vi "M2因子计算.vi"(8 "method":T1 items=["Least Square", "Least Absolute Residual", "Bisquare"], 9 "位置":dbl[](array[numeric]), 10 "光斑半径":dbl[](array[numeric]), 11 "激光波长":dbl) -> (0 "瑞利长度":dbl, 1 "束腰直径":dbl, 2 "束腰位置Z0":dbl, 3 "M2因子":dbl, 4 "光束发散角":dbl)   [LabVIEW 2015]
uses:
  <vilib>/Analysis/6fits.llb/Curve Fitting Criteria.ctl
  <vilib>/Analysis/NI_AALPro.lvlib
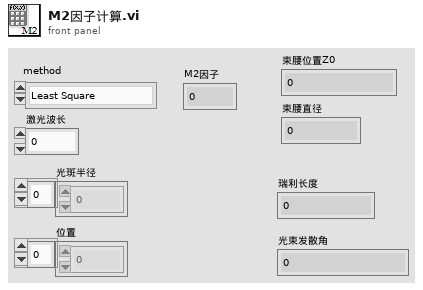
[diagram p1: front panel]
types:
  T1 = typedef "NI_AALPro.lvlib/Curve Fitting Criteria.ctl" = u16
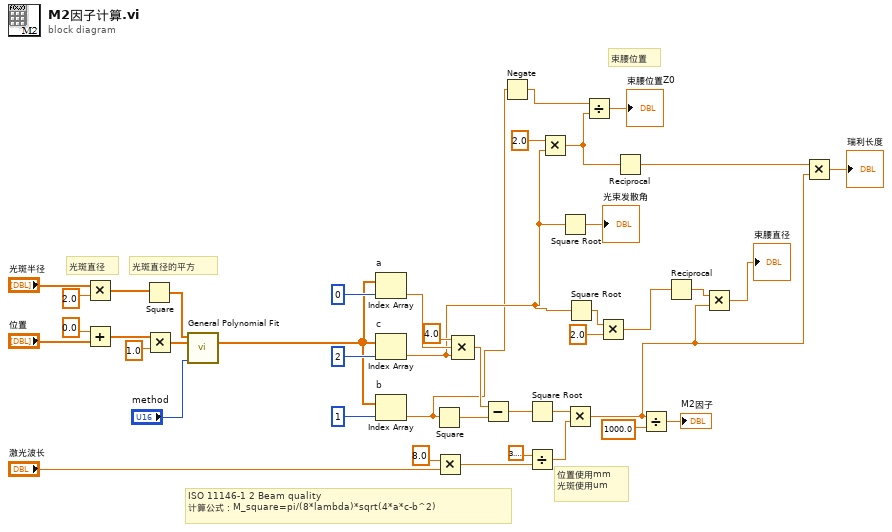
[diagram p0: block diagram]
diagram:
  # "束腰位置"
  # "位置使用mm\n光斑使用um"
  # "ISO 11146-1 2 Beam quality\n计算公式：M_square=pi/(8*lambda)*sqrt(4*a*c-b^2)"
  # "光斑直径的平方"
  # "光斑直径"
  n1 = Multiply(x="光斑半径", y=2.0) -> (x*y=w38:dbl[])
  n2 = Add(x=0.0, y="位置") -> (x+y=w41:dbl[])
  n3 = Square(x=w38) -> (x^2=w37:dbl[])
  n4 = Multiply(x=w41, y=1.0 ("x")) -> (x*y=w36:dbl[])
  n5 = call <vilib>:"General Polynomial Fit.vi"("Y"=w37, "X"=w36, "method"="method") -> ("Polynomial Coefficients"=w21:dbl[])  [unwired: 9 in, 3 out]
  n6 = Index Array "a"(array=w21, index=0) -> (element=w31:dbl)
  n7 = Index Array "c"(array=w21, index=2) -> (element=w4:dbl)
  n8 = Index Array "b"(array=w21, index=1) -> (element=w3:dbl)
  n9 = Square(x=w3) -> (x^2=w29:dbl)
  n10 = Multiply(x=8.0, y="激光波长") -> (x*y=w26:dbl)
  n11 = Compound Arithmetic op=MULTIPLY(4.0 ("value"), w31, w4) -> (w30:dbl)
  n12 = Subtract(x=w30, y=w29) -> (x-y=w28:dbl)
  n13 = Negate(x=w3) -> (-x=w9:dbl)
  n14 = Square Root(x=w28) -> (sqrt(x)=w23:dbl)
  n15 = Divide(x=3.141592653589793, y=w26) -> (x/y=w24:dbl)
  n16 = Multiply(x=2.0, y=w4) -> (x*y=w13:dbl)
  n17 = Square Root(x=w4) -> (sqrt(x)=→"光束发散角":dbl)
  n18 = Multiply(x=w23, y=w24) -> (x*y=w1:dbl)
  n19 = Square Root(x=w4) -> (sqrt(x)=w5:dbl)
  n20 = Divide(x=w9, y=w13) -> (x/y=→"束腰位置Z0":dbl)
  n21 = Multiply(x=w5, y=2.0) -> (x*y=w7:dbl)
  n22 = Reciprocal(x=w13) -> (1/x=w14:dbl)
  n23 = Divide(x=w1, y=1000.0) -> (x/y=→"M2因子":dbl)
  n24 = Reciprocal(x=w7) -> (1/x=w8:dbl)
  n25 = Multiply(x=w8, y=w1) -> (x*y=→"束腰直径":dbl)
  n26 = Multiply(x=w14, y=w1) -> (x*y=→"瑞利长度":dbl)
